vi "offset.vi"(10 "offsetChars":cluster{"Horizontal":dbl, "Vertical":dbl}, 11 "String in":string) -> (3 "String out":string)   [LabVIEW 2013]
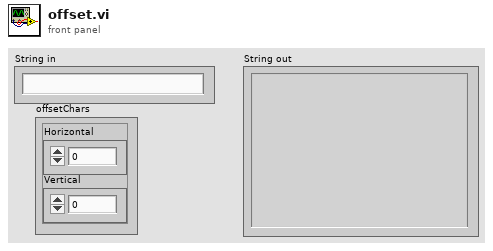
[diagram p1: front panel]
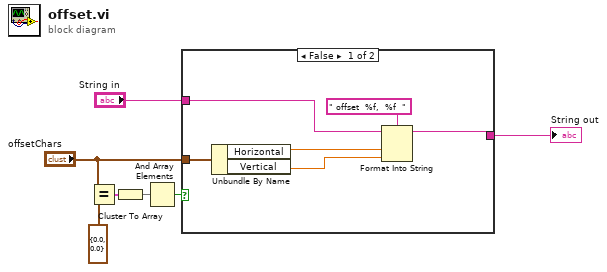
[diagram p0: block diagram]
diagram:
  n1 = Equal?(x="offsetChars", y=cluster{"Horizontal":dbl, "Vertical":dbl} {"Horizontal"=0.0, "Vertical"=0.0} ("offsetChars")) -> (x = y?=w2:cluster{"Horizontal":bool, "Vertical":bool})
  n2 = Cluster To Array(cluster=w2) -> (array=w1:bool[])
  n3 = And Array Elements(Boolean array=w1) -> (logical AND=w3:bool)
  n4 = case shown="False" w3 {
    tunnel: [w13 w14] -> w7
    tunnel: "String in" -> [w12 w14]
    tunnel: "offsetChars" -> [w8 _]
    frame False {
      n5 = Unbundle By Name(w8) -> ("Horizontal"=w10:dbl, "Vertical"=w9:dbl)
      n6 = Format Into String(format string=" offset  %f,  %f  ", initial string=w12, w10, w9) -> (resulting string=w13:string)  [unwired: 1 in, 1 out]
    }
    frame True {
    }
  }
  "String out" <- w7
